vi "Obtain Broadcast Events for Registration.vi"(8 "error in":errorcluster) -> (0 "error out":errorcluster, 2 "Already running?":bool, 3 "EL72xxDMC_Drive Broadcast Events":T1)   [LabVIEW 2023, in "EL72xxDMC_Drive.lvlib"]
doc: "Return the broadcast event refnums so the module's caller can register for the module's broadcast events.\n_____\nBased on DQMH Project Template 7.0.1.1316."
uses:
  EL72xxDMC_Drive.lvlib
  Broadcast Events--cluster.ctl
  Did Init Argument--cluster.ctl
  Status Updated Argument--cluster.ctl
  Error Reported Argument--cluster.ctl
  Stop Argument--cluster.ctl
  Get Module Execution Status Argument--cluster.ctl
  Module Running State--enum.ctl
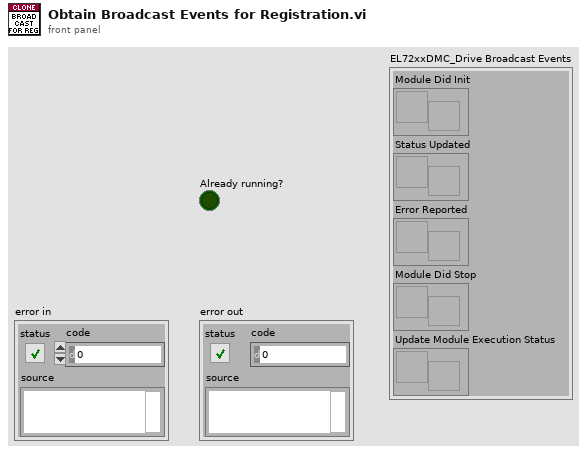
[diagram p1: front panel]
types:
  T1 = typedef "EL72xxDMC_Drive.lvlib/Broadcast Events--cluster.ctl" = cluster{"Module Did Init":refnum<user-event>, "Status Updated":refnum<user-event>, "Error Reported":refnum<user-event>, "Module Did Stop":refnum<user-event>, "Update Module Execution Status":refnum<user-event>}
  T2 = typedef "EL72xxDMC_Drive.lvlib/Module Running State--enum.ctl" = enum16{"Not Running", "Running as Cloneable", "Running as Singleton"}
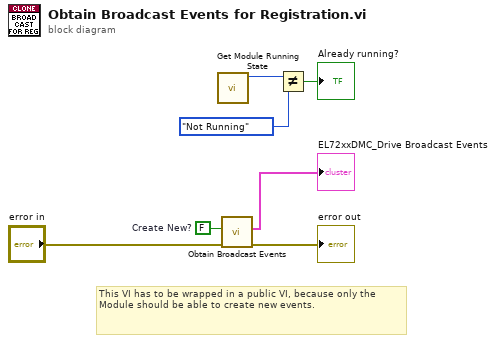
[diagram p0: block diagram]
diagram:
  w5 = FALSE  # Create New?
  # "This VI has to be wrapped in a public VI, because only the Module should be able to create new events."
  n1 = call "Get Module Running State.vi"() -> ("Module Running State"=w3:T2)  [unwired: 11 in]
  n2 = call "Obtain Broadcast Events.vi"("error in"="error in", "Create New? (F)"=w5) -> ("error out"=→"error out":errorcluster, "EL72xxDMC_Drive Broadcast Events"=→"EL72xxDMC_Drive Broadcast Events":T1)  [unwired: 8 in]
  n3 = Not Equal?(x=w3, y=Module_Running_State--enum."Not Running") -> (x != y?=→"Already running?":bool)
